vi "AlGaInPAs_v19b.vi"(2 "Debug Mode":bool, 3 "Elapsed Time(s)":dbl, 4 "State":enum16{"Edit", "Start", "Run", "End", "Idle"}(ring), 5 "Argument List In":string[](array[string])) -> (0 "Status Out":string, 1 "Argument List Out":string[](array[string]))   [LabVIEW 2011]
panel:
  out "In bubbler":T1 {"In main Copy"."Flow" format="%.2f"}
  out "Al bubbler":T2 {"Al main Copy"."Al Flow" format="%.2f"}
  out "P bubbler":T3 {"P bubbler main Copy"."Flow" format="%.2f"}
  out "As gas":T4 {"As gas main Copy"."Flow" format="%.2f"}
  out "P gas":T5 {"P gas main Copy"."Flow" format="%.2f"}
  out "Ga Bubbler":T6={"Ga main copy"={"Flow"=0.0, "Run"=FALSE, "Prep Ga"=FALSE, "Dilution"=FALSE}, "Ga MFC Flows copy"={"MFC2 flow"=10.0, "MFC3 flow"=100.0, "MFC1 flow"=1.0}, "Ga Calculated Copy"=1, "Ga bubbler Active"=FALSE} {"Ga Calculated Copy" items=["Ga flow", "MFC1", "MFC2", "MFC3"]; "Ga MFC Flows copy"."MFC1 flow" format="%.4f"; "Ga MFC Flows copy"."MFC3 flow" format="%.1f"; "Ga MFC Flows copy"."MFC2 flow" format="%.2f"; "Ga main copy"."Flow" format="%.2f"}
  in  "Al main":T7 caption="Al" {"Al Flow" format="%.2f"}
  in  "As gas main":T8 caption="Al" {"Flow" format="%.2f"}
  in  "P bubbler main":cluster{"Flow":dbl, "Run":bool, "Prep":bool} caption="Al" {"Flow" format="%.2f"}
  in  "P gas main":cluster{"Flow":dbl, "Run":bool, "Prep":bool} caption="Al" {"Flow" format="%.2f"}
  in  "In main":cluster{"Flow":dbl, "Run":bool, "Prep In":bool} caption="Al" {"Flow" format="%.2f"}
  out "prep_done":bool
  out "run started":bool
  out "first":bool=TRUE
  out "total time":dbl
  out "is OK?":bool
  in  "prep_time":dbl
  in  "Cancel":bool
  in  "OK":bool
  out "tTotal(s) 2":dbl
  in  "Ga Tab Control":enum32{"Page 1", "Page 2", "Page 3"}(tab)
  in  "Ga main":T9 caption="Al" {"Flow" format="%.2f"}
  in  "Ga MFC Flows":T10={"MFC2 flow"=10.0, "MFC3 flow"=100.0, "MFC1 flow"=1.0} {"MFC1 flow" format="%.4f"; "MFC3 flow" format="%.1f"; "MFC2 flow" format="%.2f"}
  in  "Ga Calculated":u16(ring)=1 caption="Calculated" items=["Ga flow", "MFC1", "MFC2", "MFC3"]
  # "Add pre-run time to run time in editor."
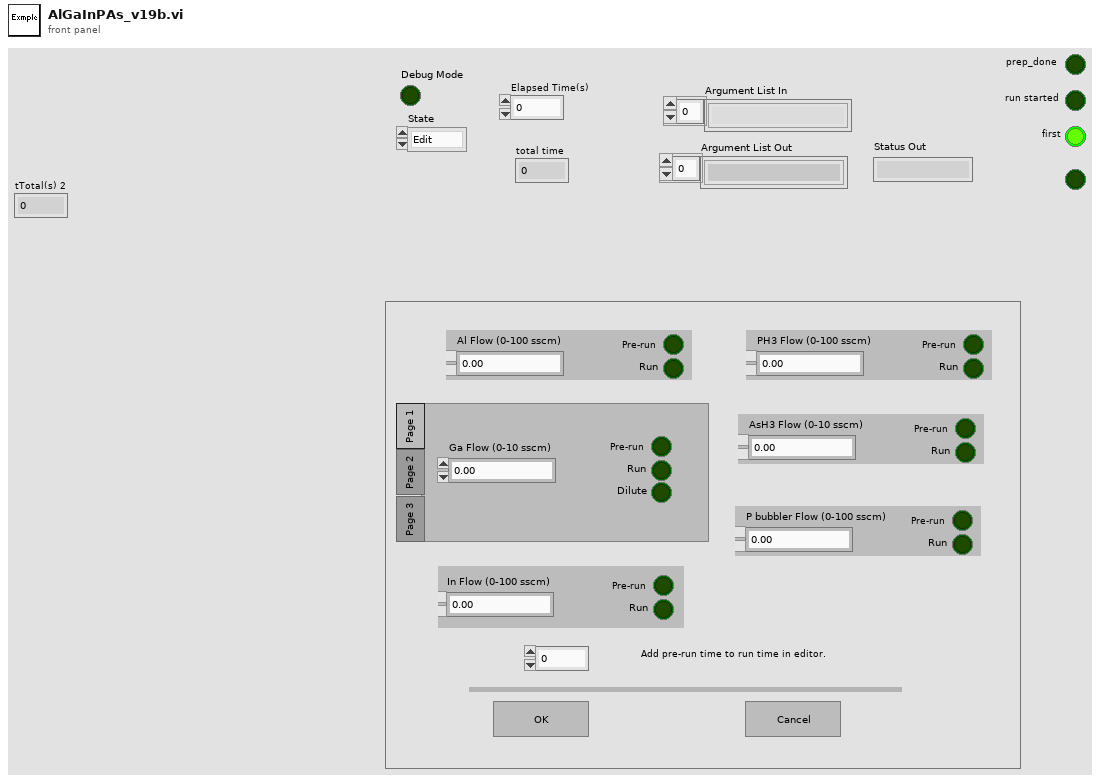
[diagram p1: front panel]
types:
  T1 = cluster{"In bubbler Active":bool, "In main Copy":cluster{"Flow":dbl, "Run":bool, "Prep In":bool}}
  T2 = cluster{"Al Active":bool, "Al main Copy":cluster{"Al Flow":dbl, "Al Run":bool, "Prep Al":bool}}
  T3 = cluster{"P bubbler Active":bool, "P bubbler main Copy":cluster{"Flow":dbl, "Run":bool, "Prep":bool}}
  T4 = cluster{"As gas Active":bool, "As gas main Copy":cluster{"Flow":dbl, "AsH3 Run":bool, "AsH3 Prep":bool}}
  T5 = cluster{"P gas Active":bool, "P gas main Copy":cluster{"Flow":dbl, "Run":bool, "Prep":bool}}
  T6 = cluster{"Ga main copy":cluster{"Flow":dbl, "Run":bool, "Prep Ga":bool, "Dilution":bool}, "Ga MFC Flows copy":cluster{"MFC2 flow":dbl, "MFC3 flow":dbl, "MFC1 flow":dbl}, "Ga Calculated Copy":u16, "Ga bubbler Active":bool}
  T7 = cluster{"Al Flow":dbl, "Al Run":bool, "Prep Al":bool}
  T8 = cluster{"Flow":dbl, "AsH3 Run":bool, "AsH3 Prep":bool}
  T9 = cluster{"Flow":dbl, "Run":bool, "Prep Ga":bool, "Dilution":bool}
  T10 = cluster{"MFC2 flow":dbl, "MFC3 flow":dbl, "MFC1 flow":dbl}
  T11 = enum16{"Discrete", "Continuous", "Instantaneous", "Finite"}
  T12 = enum32{"Invalid", "Default", "Floating", "Floating/Auto-Hide", "Modal"}
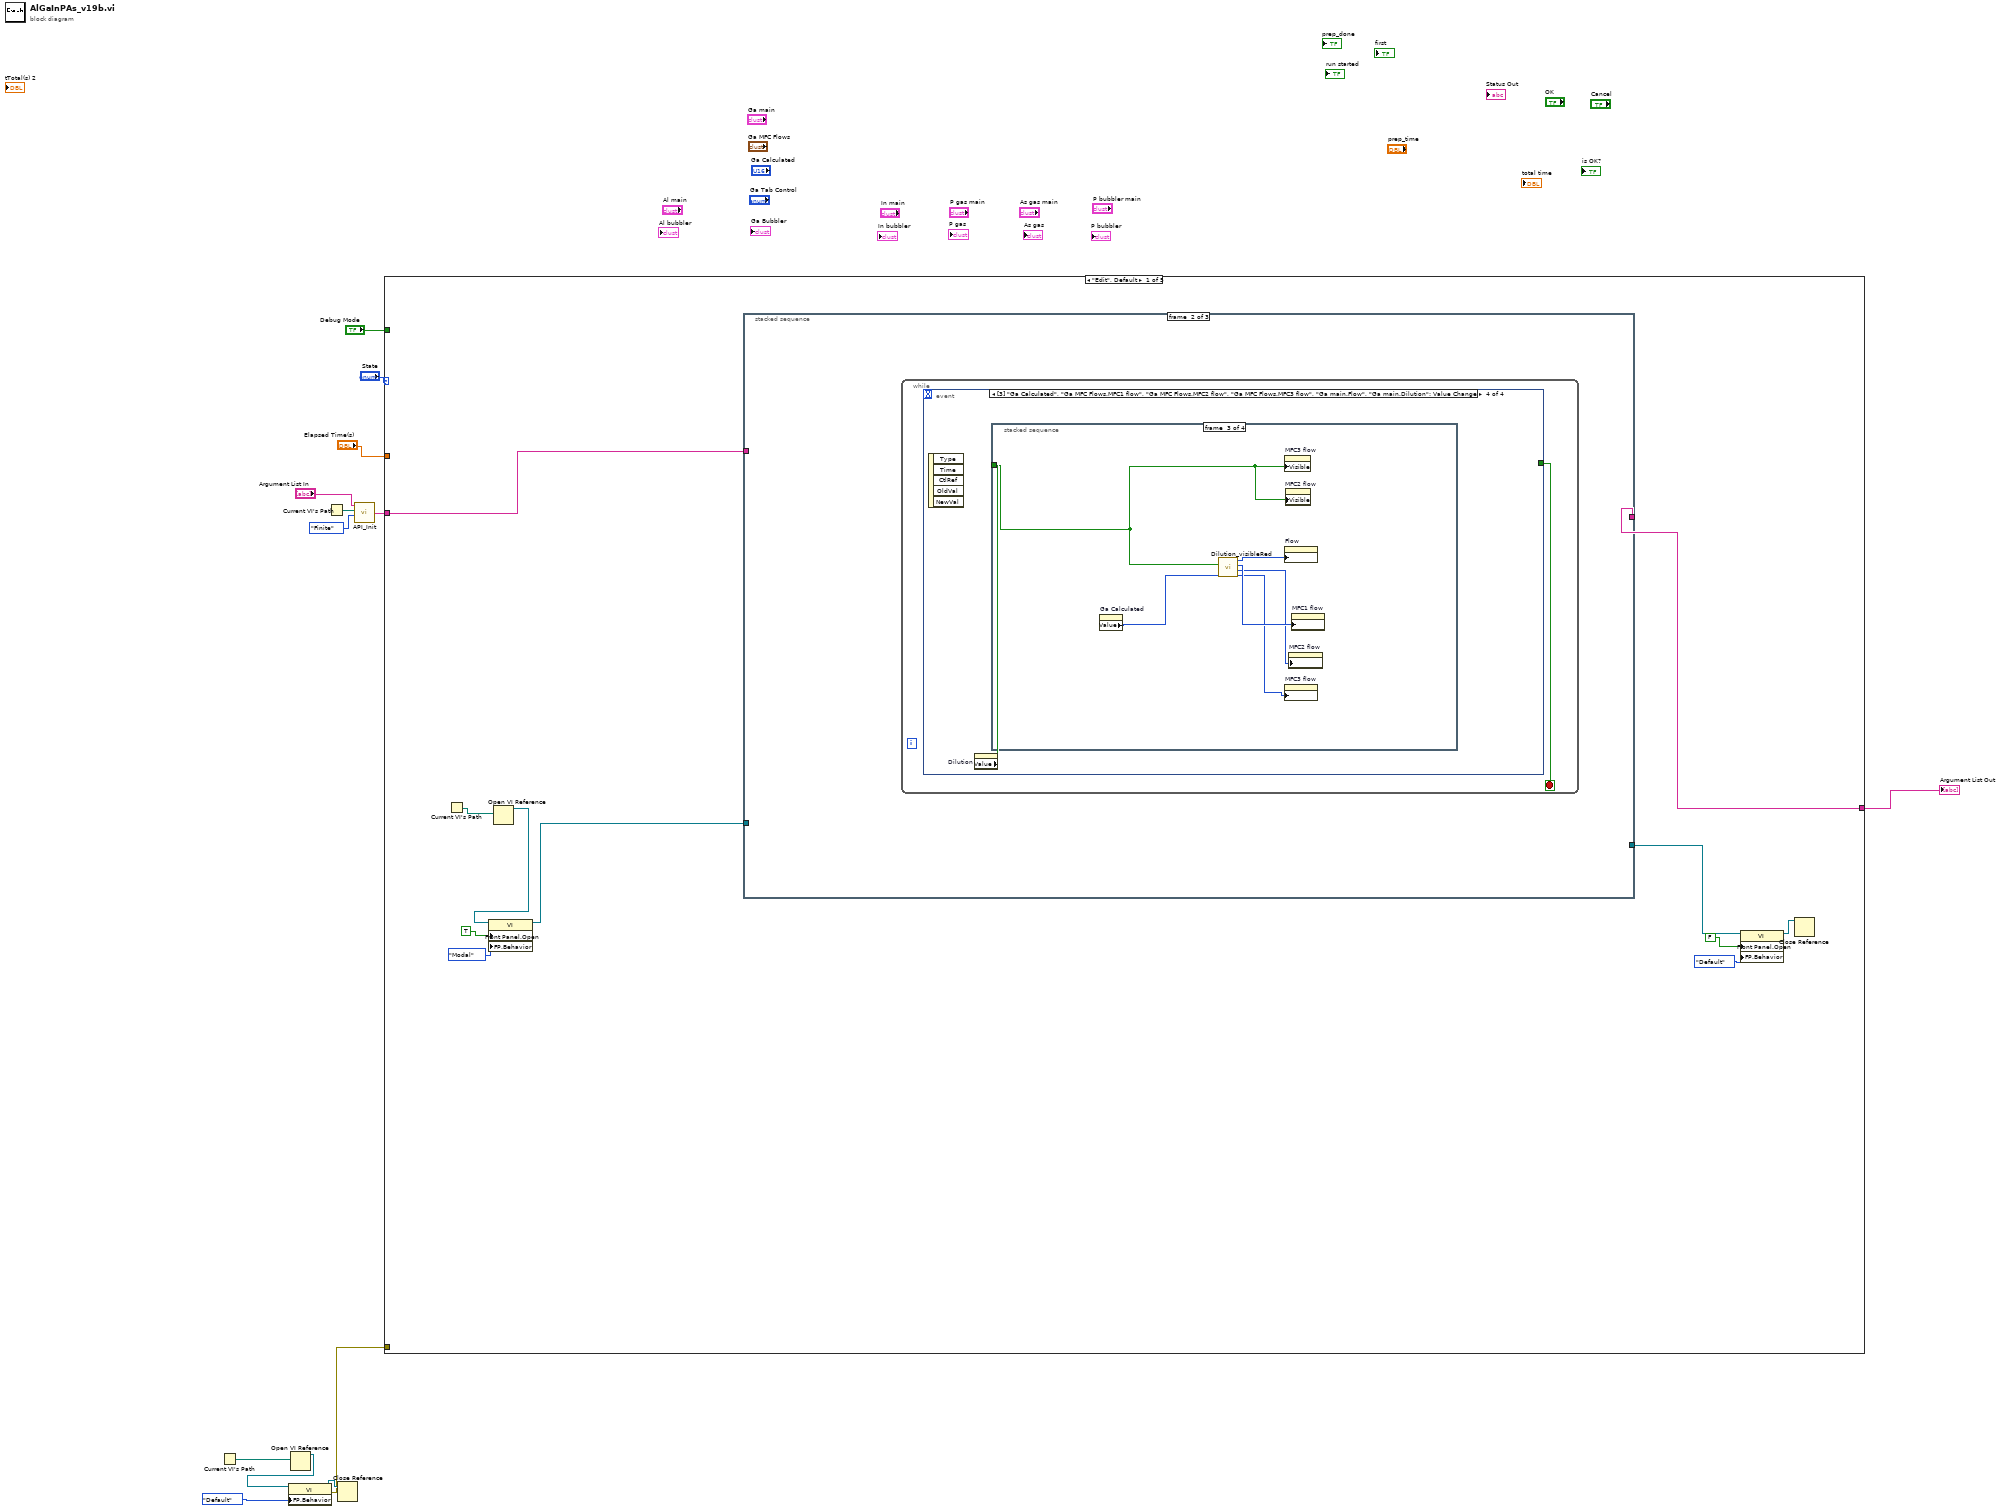
[diagram p0: block diagram]
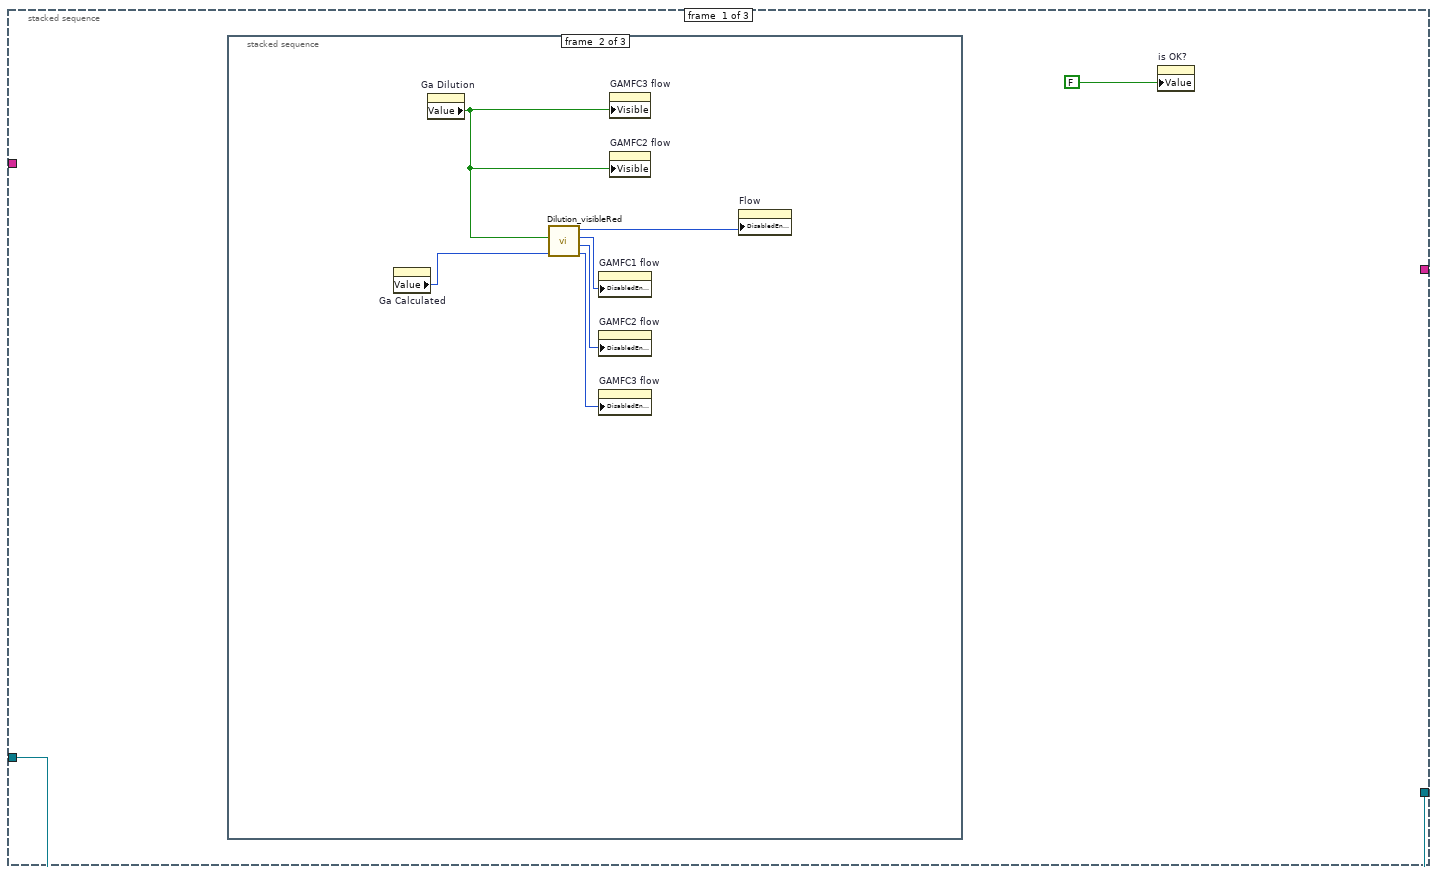
[diagram p2: hidden frame]
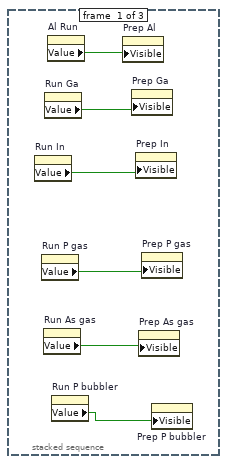
[diagram p3: hidden frame]
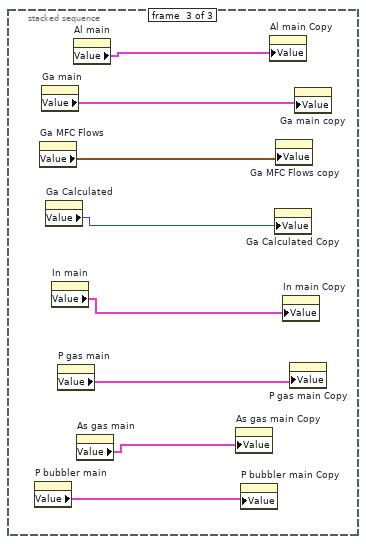
[diagram p4: hidden frame]
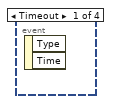
[diagram p5: hidden frame]
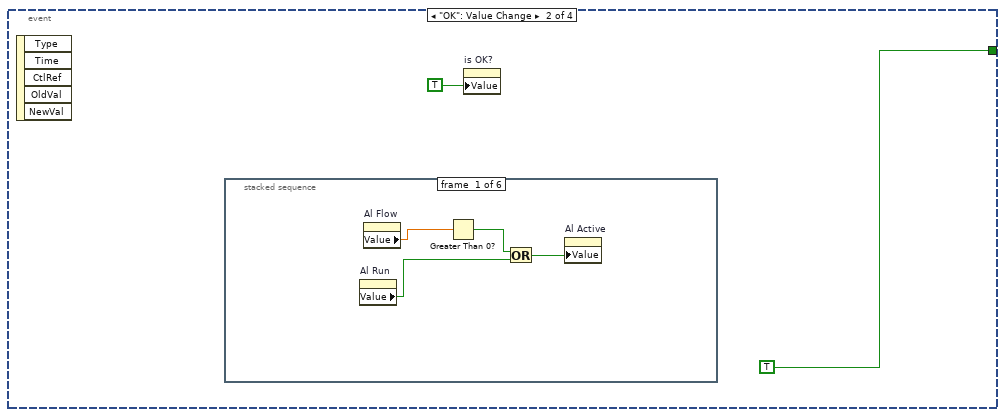
[diagram p6: hidden frame]
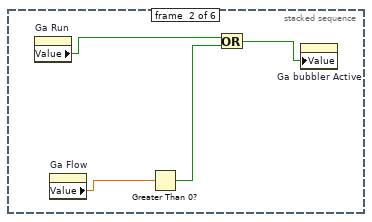
[diagram p7: hidden frame]
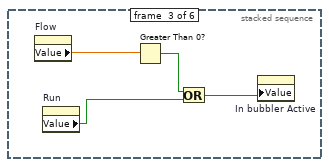
[diagram p8: hidden frame]
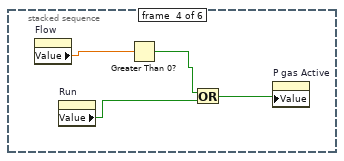
[diagram p9: hidden frame]
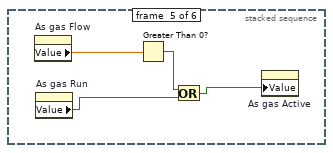
[diagram p10: hidden frame]
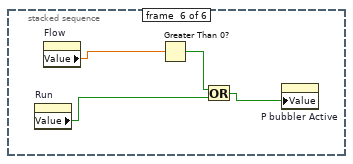
[diagram p11: hidden frame]
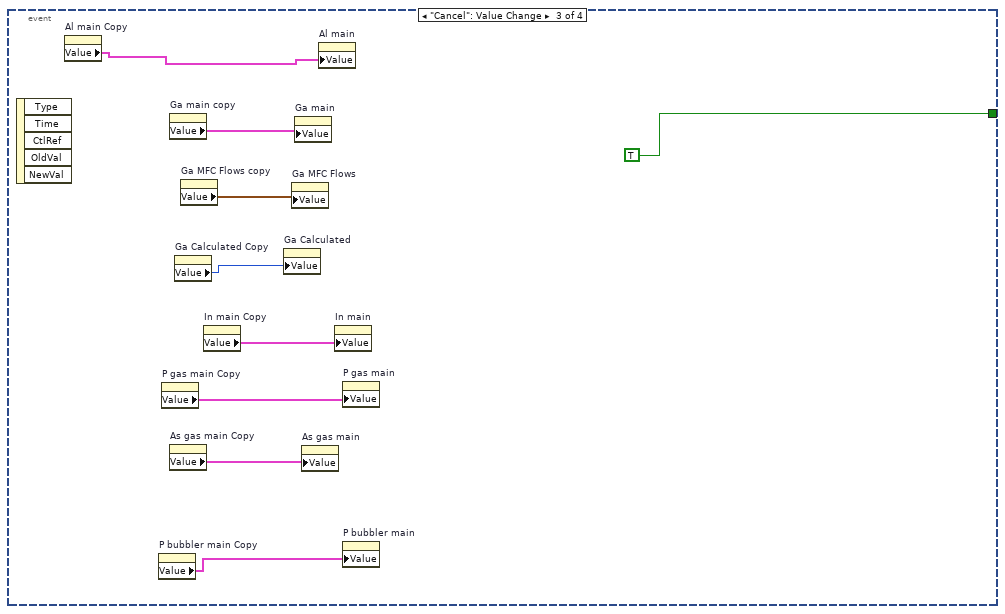
[diagram p12: hidden frame]
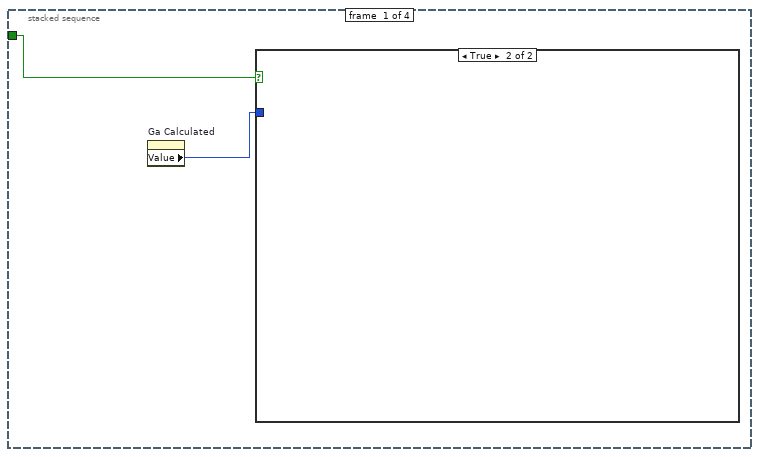
[diagram p13: hidden frame]
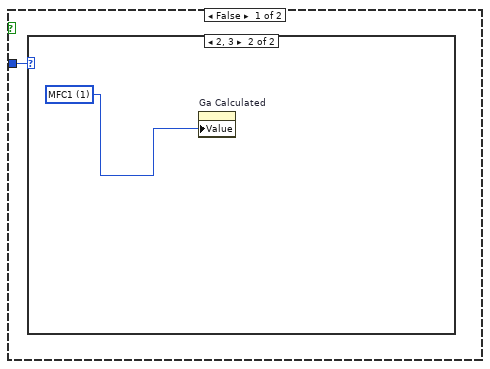
[diagram p14: hidden frame]
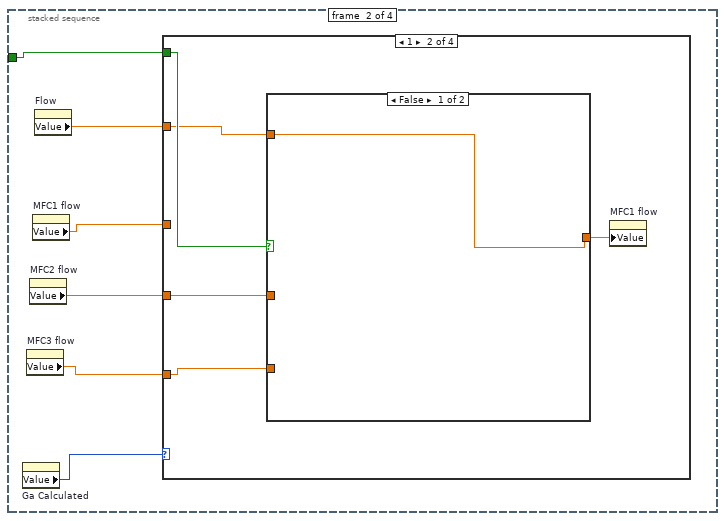
[diagram p16: hidden frame]
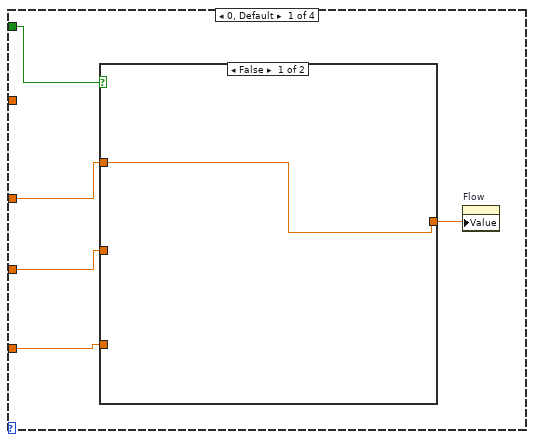
[diagram p17: hidden frame]
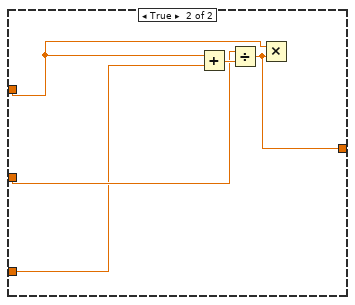
[diagram p18: hidden frame]
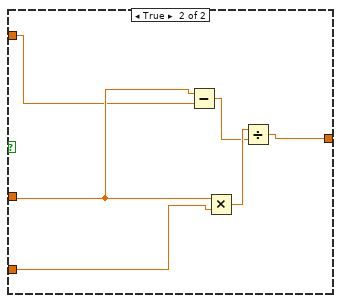
[diagram p19: hidden frame]
diagram:
  n1 = Current VI's Path() -> (path=w9:path)
  n2 = Open VI Reference(vi path=w9) -> (vi reference=w8:refnum<vi>)  [unwired: 1 in, 5 out]
  n3 = property class="VI"(reference=w8, "FP.Behavior"=T12."Default" ("Front Panel Window:Behavior")) -> (reference out=w6:refnum<vi>, error out=w5:errorcluster)  [unwired: 1 in]
  n4 = Current VI's Path() -> (path=w4:path)
  n5 = Close Reference(reference=w6) -> ()  [unwired: 1 in, 1 out]
  n6 = call "API_Init.vi"("API Mode"=T11."Finite", "VI Path"=w4, "Argument List In"="Argument List In") -> ("Argument List Out"=w1:string[])  [unwired: 1 in]
  n7 = case shown="\"Edit\", Default" "State" {
    tunnel: "Debug Mode" -> [_ w151 w209 _ _]
    tunnel: "Elapsed Time(s)" -> [_ _ w210 _ _]
    tunnel: w1 -> [w15 w153 w208 w314 w315]
    tunnel: [w14 w152 w207 w314 w315] -> w10
    tunnel: w5 -> [_ _ _ _ _]
    frame "Edit", Default {
      n8 = Current VI's Path() -> (path=w20:path)
      n9 = Open VI Reference(vi path=w20) -> (vi reference=w19:refnum<vi>)  [unwired: 1 in, 5 out]
      n10 = property class="VI"(reference=w19, "Front Panel.Open"=TRUE ("Front Panel Window:Open"), "FP.Behavior"=T12."Modal" ("Front Panel Window:Behavior")) -> (reference out=w18:refnum<vi>)  [unwired: 1 in, 1 out]
      n11 = stacked-sequence {
        tunnel: w15 -> [_ _ w147]
        tunnel: w18 -> [w26 _ _]
        tunnel: [w26 _ _] -> w22
        tunnel: [_ _ w148] -> w14
        frame #0 {
          n12 = stacked-sequence {
            frame #0 {
              n13 = property on="Run In" class="Bool (strict)"() -> ("Value"=w31:bool)  [unwired: 2 in, 2 out]
              n14 = property on="Run P gas" class="Bool (strict)"() -> ("Value"=w29:bool)  [unwired: 2 in, 2 out]
              n15 = property on="Run As gas" class="Bool (strict)"() -> ("Value"=w28:bool)  [unwired: 2 in, 2 out]
              n16 = property on="Run Ga" class="Bool (strict)"() -> ("Value"=w30:bool)  [unwired: 2 in, 2 out]
              n17 = property on="Al Run" class="Bool (strict)"() -> ("Value"=w32:bool)  [unwired: 2 in, 2 out]
              n18 = property on="Run P bubbler" class="Bool (strict)"() -> ("Value"=w27:bool)  [unwired: 2 in, 2 out]
              n19 = property on="Prep Al" class="Bool (strict)"("Visible"=w32) -> ()  [unwired: 2 in, 2 out]
              n20 = property on="Prep Ga" class="Bool (strict)"("Visible"=w30) -> ()  [unwired: 2 in, 2 out]
              n21 = property on="Prep In" class="Bool (strict)"("Visible"=w31) -> ()  [unwired: 2 in, 2 out]
              n22 = property on="Prep As gas" class="Bool (strict)"("Visible"=w28) -> ()  [unwired: 2 in, 2 out]
              n23 = property on="Prep P gas" class="Bool (strict)"("Visible"=w29) -> ()  [unwired: 2 in, 2 out]
              n24 = property on="Prep P bubbler" class="Bool (strict)"("Visible"=w27) -> ()  [unwired: 2 in, 2 out]
            }
            frame #1 {
              n25 = property on="Ga Calculated" class="Ring (strict)"() -> ("Value"=w38:u16)  [unwired: 2 in, 2 out]
              n26 = property on="Ga Dilution" class="Bool (strict)"() -> ("Value"=w37:bool)  [unwired: 2 in, 2 out]
              n27 = call "Dilution_visibleRed.vi"("calculated"=w38, "dilution"=w37) -> ("MFC3"=w34:u16, "MFC2"=w35:u16, "MFC1"=w36:u16, "flow"=w33:u16)  [unwired: 2 in]
              n28 = property on="GAMFC1 flow" class="DigNum (strict)"("DisabledEnum"=w36) -> ()  [unwired: 2 in, 2 out]
              n29 = property on="GAMFC2 flow" class="DigNum (strict)"("DisabledEnum"=w35) -> ()  [unwired: 2 in, 2 out]
              n30 = property on="GAMFC3 flow" class="DigNum (strict)"("DisabledEnum"=w34) -> ()  [unwired: 2 in, 2 out]
              n31 = property on="GAMFC3 flow" class="DigNum (strict)"("Visible"=w37) -> ()  [unwired: 2 in, 2 out]
              n32 = property on="GAMFC2 flow" class="DigNum (strict)"("Visible"=w37) -> ()  [unwired: 2 in, 2 out]
              n33 = property on="Flow" class="DigNum (strict)"("DisabledEnum"=w33) -> ()  [unwired: 2 in, 2 out]
            }
            frame #2 {
              n34 = property on="P bubbler main" class="Clust (strict)"() -> ("Value"=w40:cluster{"Flow":dbl, "Run":bool, "Prep":bool})  [unwired: 2 in, 2 out]
              n35 = property on="Ga MFC Flows" class="Clust (strict)"() -> ("Value"=w45:T10)  [unwired: 2 in, 2 out]
              n36 = property on="Ga main" class="Clust (strict)"() -> ("Value"=w46:T9)  [unwired: 2 in, 2 out]
              n37 = property on="Ga Calculated" class="Ring (strict)"() -> ("Value"=w44:u16)  [unwired: 2 in, 2 out]
              n38 = property on="In main" class="Clust (strict)"() -> ("Value"=w43:cluster{"Flow":dbl, "Run":bool, "Prep In":bool})  [unwired: 2 in, 2 out]
              n39 = property on="P gas main" class="Clust (strict)"() -> ("Value"=w42:cluster{"Flow":dbl, "Run":bool, "Prep":bool})  [unwired: 2 in, 2 out]
              n40 = property on="Al main" class="Clust (strict)"() -> ("Value"=w39:T7)  [unwired: 2 in, 2 out]
              n41 = property on="As gas main" class="Clust (strict)"() -> ("Value"=w41:T8)  [unwired: 2 in, 2 out]
              n42 = property on="As gas main Copy" class="Clust (strict)"("Value"=w41) -> ()  [unwired: 2 in, 2 out]
              n43 = property on="P bubbler main Copy" class="Clust (strict)"("Value"=w40) -> ()  [unwired: 2 in, 2 out]
              n44 = property on="Al main Copy" class="Clust (strict)"("Value"=w39) -> ()  [unwired: 2 in, 2 out]
              n45 = property on="Ga Calculated Copy" class="Ring (strict)"("Value"=w44) -> ()  [unwired: 2 in, 2 out]
              n46 = property on="Ga MFC Flows copy" class="Clust (strict)"("Value"=w45) -> ()  [unwired: 2 in, 2 out]
              n47 = property on="In main Copy" class="Clust (strict)"("Value"=w43) -> ()  [unwired: 2 in, 2 out]
              n48 = property on="P gas main Copy" class="Clust (strict)"("Value"=w42) -> ()  [unwired: 2 in, 2 out]
              n49 = property on="Ga main copy" class="Clust (strict)"("Value"=w46) -> ()  [unwired: 2 in, 2 out]
            }
          }
          n50 = property on="is OK?" class="Bool (strict)"("Value"=FALSE ("is OK?")) -> ()  [unwired: 2 in, 2 out]
        }
        frame #1 {
          n51 = while {
            stop <- w47 stop-if-true
            n52 = event shown="[3] \"Ga Calculated\", \"Ga MFC Flows.MFC1 flow\", \"Ga MFC Flows.MFC2 flow\", \"Ga MFC Flows.MFC3 flow\", \"Ga main.Flow\", \"Ga main.Dilution\": Value Change" {
              selector: _ -> [_ _ _ _]
              dyn-events: _ -> [_ _ _ _]
              timeout: _ -> [_ _ _ _]
              tunnel: [_ TRUE TRUE _] -> w47
              event Timeout {
                n53 = event-data() -> ()  [unwired: 1 in, 2 out]
              }
              event "OK": Value Change {
                n54 = event-data() -> ()  [unwired: 1 in, 5 out]
                n55 = stacked-sequence {
                  frame #0 {
                    n56 = property on="Al Run" class="Bool (strict)"() -> ("Value"=w51:bool)  [unwired: 2 in, 2 out]
                    n57 = property on="Al Flow" class="DigNum (strict)"() -> ("Value"=w52:dbl)  [unwired: 2 in, 2 out]
                    n58 = Greater Than 0?(x=w52) -> (x > 0?=w53:bool)
                    n59 = Or(x=w53, y=w51) -> (x .or. y?=w50:bool)
                    n60 = property on="Al Active" class="Bool (strict)"("Value"=w50) -> ()  [unwired: 2 in, 2 out]
                  }
                  frame #1 {
                    n61 = property on="Ga Run" class="Bool (strict)"() -> ("Value"=w55:bool)  [unwired: 2 in, 2 out]
                    n62 = property on="Ga Flow" class="DigNum (strict)"() -> ("Value"=w54:dbl)  [unwired: 2 in, 2 out]
                    n63 = Greater Than 0?(x=w54) -> (x > 0?=w57:bool)
                    n64 = Or(x=w55, y=w57) -> (x .or. y?=w56:bool)
                    n65 = property on="Ga bubbler Active" class="Bool (strict)"("Value"=w56) -> ()  [unwired: 2 in, 2 out]
                  }
                  frame #2 {
                    n66 = property on="Flow" class="DigNum (strict)"() -> ("Value"=w60:dbl)  [unwired: 2 in, 2 out]
                    n67 = property on="Run" class="Bool (strict)"() -> ("Value"=w59:bool)  [unwired: 2 in, 2 out]
                    n68 = Greater Than 0?(x=w60) -> (x > 0?=w61:bool)
                    n69 = Or(x=w61, y=w59) -> (x .or. y?=w58:bool)
                    n70 = property on="In bubbler Active" class="Bool (strict)"("Value"=w58) -> ()  [unwired: 2 in, 2 out]
                  }
                  frame #3 {
                    n71 = property on="Flow" class="DigNum (strict)"() -> ("Value"=w64:dbl)  [unwired: 2 in, 2 out]
                    n72 = property on="Run" class="Bool (strict)"() -> ("Value"=w63:bool)  [unwired: 2 in, 2 out]
                    n73 = Greater Than 0?(x=w64) -> (x > 0?=w65:bool)
                    n74 = Or(x=w65, y=w63) -> (x .or. y?=w62:bool)
                    n75 = property on="P gas Active" class="Bool (strict)"("Value"=w62) -> ()  [unwired: 2 in, 2 out]
                  }
                  frame #4 {
                    n76 = property on="As gas Flow" class="DigNum (strict)"() -> ("Value"=w68:dbl)  [unwired: 2 in, 2 out]
                    n77 = property on="As gas Run" class="Bool (strict)"() -> ("Value"=w67:bool)  [unwired: 2 in, 2 out]
                    n78 = Greater Than 0?(x=w68) -> (x > 0?=w69:bool)
                    n79 = Or(x=w69, y=w67) -> (x .or. y?=w66:bool)
                    n80 = property on="As gas Active" class="Bool (strict)"("Value"=w66) -> ()  [unwired: 2 in, 2 out]
                  }
                  frame #5 {
                    n81 = property on="Run" class="Bool (strict)"() -> ("Value"=w71:bool)  [unwired: 2 in, 2 out]
                    n82 = property on="Flow" class="DigNum (strict)"() -> ("Value"=w72:dbl)  [unwired: 2 in, 2 out]
                    n83 = Greater Than 0?(x=w72) -> (x > 0?=w73:bool)
                    n84 = Or(x=w73, y=w71) -> (x .or. y?=w70:bool)
                    n85 = property on="P bubbler Active" class="Bool (strict)"("Value"=w70) -> ()  [unwired: 2 in, 2 out]
                  }
                }
                n86 = property on="is OK?" class="Bool (strict)"("Value"=TRUE ("is OK?")) -> ()  [unwired: 2 in, 2 out]
              }
              event "Cancel": Value Change {
                n87 = event-data() -> ()  [unwired: 1 in, 5 out]
                n88 = property on="Al main Copy" class="Clust (strict)"() -> ("Value"=w74:T7)  [unwired: 2 in, 2 out]
                n89 = property on="P bubbler main Copy" class="Clust (strict)"() -> ("Value"=w75:cluster{"Flow":dbl, "Run":bool, "Prep":bool})  [unwired: 2 in, 2 out]
                n90 = property on="P gas main Copy" class="Clust (strict)"() -> ("Value"=w80:cluster{"Flow":dbl, "Run":bool, "Prep":bool})  [unwired: 2 in, 2 out]
                n91 = property on="Ga main copy" class="Clust (strict)"() -> ("Value"=w79:T9)  [unwired: 2 in, 2 out]
                n92 = property on="As gas main Copy" class="Clust (strict)"() -> ("Value"=w76:T8)  [unwired: 2 in, 2 out]
                n93 = property on="Ga Calculated Copy" class="Ring (strict)"() -> ("Value"=w77:u16)  [unwired: 2 in, 2 out]
                n94 = property on="Ga MFC Flows copy" class="Clust (strict)"() -> ("Value"=w78:T10)  [unwired: 2 in, 2 out]
                n95 = property on="In main Copy" class="Clust (strict)"() -> ("Value"=w81:cluster{"Flow":dbl, "Run":bool, "Prep In":bool})  [unwired: 2 in, 2 out]
                n96 = property on="Ga Calculated" class="Ring (strict)"("Value"=w77) -> ()  [unwired: 2 in, 2 out]
                n97 = property on="Ga MFC Flows" class="Clust (strict)"("Value"=w78) -> ()  [unwired: 2 in, 2 out]
                n98 = property on="Ga main" class="Clust (strict)"("Value"=w79) -> ()  [unwired: 2 in, 2 out]
                n99 = property on="As gas main" class="Clust (strict)"("Value"=w76) -> ()  [unwired: 2 in, 2 out]
                n100 = property on="Al main" class="Clust (strict)"("Value"=w74) -> ()  [unwired: 2 in, 2 out]
                n101 = property on="In main" class="Clust (strict)"("Value"=w81) -> ()  [unwired: 2 in, 2 out]
                n102 = property on="P gas main" class="Clust (strict)"("Value"=w80) -> ()  [unwired: 2 in, 2 out]
                n103 = property on="P bubbler main" class="Clust (strict)"("Value"=w75) -> ()  [unwired: 2 in, 2 out]
              }
              event "Ga Calculated", "Ga MFC Flows.MFC1 flow", "Ga MFC Flows.MFC2 flow", "Ga MFC Flows.MFC3 flow", "Ga main.Flow", "Ga main.Dilution": Value Change {
                n104 = event-data() -> ()  [unwired: 1 in, 5 out]
                n105 = property on="Dilution" class="Bool (strict)"() -> ("Value"=w83:bool)  [unwired: 2 in, 2 out]
                n106 = stacked-sequence {
                  tunnel: w83 -> [w84 w92 w137 w143]
                  frame #0 {
                    n107 = property on="Ga Calculated" class="Ring (strict)"() -> ("Value"=w85:u16)  [unwired: 2 in, 2 out]
                    n108 = case shown="True" w84 {
                      tunnel: w85 -> [w86 _]
                      frame False {
                        n109 = case shown="2, 3" w86 {
                          frame 0, 1, Default {
                          }
                          frame 2, 3 {
                            w87 = u16 1 items=["Ga flow", "MFC1", "MFC2", "MFC3"] ("Ga calculated")
                            n110 = property on="Ga Calculated" class="Ring (strict)"("Value"=w87) -> ()  [unwired: 2 in, 2 out]
                          }
                        }
                      }
                      frame True {
                      }
                    }
                  }
                  frame #1 {
                    n111 = property on="Ga Calculated" class="Ring (strict)"() -> ("Value"=w93:u16)  [unwired: 2 in, 2 out]
                    n112 = property on="MFC3 flow" class="DigNum (strict)"() -> ("Value"=w89:dbl)  [unwired: 2 in, 2 out]
                    n113 = property on="MFC2 flow" class="DigNum (strict)"() -> ("Value"=w90:dbl)  [unwired: 2 in, 2 out]
                    n114 = property on="MFC1 flow" class="DigNum (strict)"() -> ("Value"=w91:dbl)  [unwired: 2 in, 2 out]
                    n115 = property on="Flow" class="DigNum (strict)"() -> ("Value"=w88:dbl)  [unwired: 2 in, 2 out]
                    n116 = case shown="1" w93 {
                      tunnel: w92 -> [w98 w109 w120 w130]
                      tunnel: w91 -> [w97 _ w119 w129]
                      tunnel: w90 -> [w96 w106 _ w127]
                      tunnel: w89 -> [w95 w105 w118 _]
                      tunnel: w88 -> [_ w108 w117 w128]
                      frame 0, Default {
                        n117 = case shown="False" w98 {
                          tunnel: w97 -> [w99 w103]
                          tunnel: w96 -> [_ w102]
                          tunnel: w95 -> [_ w101]
                          tunnel: [w99 w100] -> w94
                          frame False {
                          }
                          frame True {
                            n118 = Add(x=w103, y=w101) -> (x+y=w104:dbl)
                            n119 = Divide(x=w102, y=w104) -> (x/y=w100:dbl)
                            n120 = Multiply(x=w103, y=w100) -> ()  [unwired: 1 out]
                          }
                        }
                        n121 = property on="Flow" class="DigNum (strict)"("Value"=w94) -> ()  [unwired: 2 in, 2 out]
                      }
                      frame 1 {
                        n122 = case shown="False" w109 {
                          tunnel: w108 -> [w110 w112]
                          tunnel: [w110 w111] -> w107
                          tunnel: w106 -> [_ w114]
                          tunnel: w105 -> [_ w113]
                          frame False {
                          }
                          frame True {
                            n123 = Subtract(x=w114, y=w112) -> (x-y=w115:dbl)
                            n124 = Multiply(x=w114, y=w113) -> (x*y=w116:dbl)
                            n125 = Divide(x=w116, y=w115) -> (x/y=w111:dbl)
                          }
                        }
                        n126 = property on="MFC1 flow" class="DigNum (strict)"("Value"=w107) -> ()  [unwired: 2 in, 2 out]
                      }
                      frame 2 {
                        n127 = case shown="False" w120 {
                          tunnel: w119 -> [_ w122]
                          tunnel: w118 -> [_ w124]
                          tunnel: w117 -> [_ w123]
                          frame False {
                          }
                          frame True {
                            n128 = Add(x=w122, y=w124) -> (x+y=w126:dbl)
                            n129 = Multiply(x=w123, y=w126) -> (x*y=w125:dbl)
                            n130 = Divide(x=w125, y=w122) -> (x/y=w121:dbl)
                            n131 = property on="MFC2 flow" class="DigNum (strict)"("Value"=w121) -> ()  [unwired: 2 in, 2 out]
                          }
                        }
                      }
                      frame 3 {
                        n132 = case shown="False" w130 {
                          tunnel: w129 -> [_ w134]
                          tunnel: w128 -> [_ w133]
                          tunnel: w127 -> [_ w132]
                          frame False {
                          }
                          frame True {
                            n133 = Subtract(x=w132, y=w133) -> (x-y=w135:dbl)
                            n134 = Divide(x=w134, y=w133) -> (x/y=w136:dbl)
                            n135 = Multiply(x=w136, y=w135) -> (x*y=w131:dbl)
                            n136 = property on="MFC3 flow" class="DigNum (strict)"("Value"=w131) -> ()  [unwired: 2 in, 2 out]
                          }
                        }
                      }
                    }
                  }
                  frame #2 {
                    n137 = property on="Ga Calculated" class="Ring (strict)"() -> ("Value"=w142:u16)  [unwired: 2 in, 2 out]
                    n138 = call "Dilution_visibleRed.vi"("calculated"=w142, "dilution"=w137) -> ("MFC3"=w138:u16, "MFC2"=w139:u16, "MFC1"=w140:u16, "flow"=w141:u16)  [unwired: 2 in]
                    n139 = property on="MFC3 flow" class="DigNum (strict)"("Visible"=w137) -> ()  [unwired: 2 in, 2 out]
                    n140 = property on="Flow" class="DigNum (strict)"("DisabledEnum"=w141) -> ()  [unwired: 2 in, 2 out]
                    n141 = property on="MFC3 flow" class="DigNum (strict)"("DisabledEnum"=w138) -> ()  [unwired: 2 in, 2 out]
                    n142 = property on="MFC2 flow" class="DigNum (strict)"("Visible"=w137) -> ()  [unwired: 2 in, 2 out]
                    n143 = property on="MFC2 flow" class="DigNum (strict)"("DisabledEnum"=w139) -> ()  [unwired: 2 in, 2 out]
                    n144 = property on="MFC1 flow" class="DigNum (strict)"("DisabledEnum"=w140) -> ()  [unwired: 2 in, 2 out]
                  }
                  frame #3 {
                    n145 = case shown="True" w143 {
                      frame False {
                        n146 = property on="Ga Calculated" class="Ring (strict)"("Disabled Items []"=i32[] [2, 3]) -> ()  [unwired: 2 in, 2 out]
                      }
                      frame True {
                        n147 = property on="Ga Calculated" class="Ring (strict)"("Disabled Items []"=i32[] []) -> ()  [unwired: 2 in, 2 out]
                      }
                    }
                  }
                }
              }
            }
          }
        }
        frame #2 {
          n148 = property on="is OK?" class="Bool (strict)"() -> ("Value"=w146:bool)  [unwired: 2 in, 2 out]
          n149 = Not(x=w146) -> (.not. x?=w150:bool)
          n150 = Current VI's Path() -> (path=w149:path)
          n151 = call "API_Edit.vi"("Cancel"=w150, "OK"=w146, "VI Path"=w149, "Argument List In"=w147) -> ("Argument List Out"=w148:string[])
        }
      }
      n152 = property class="VI"(reference=w22, "Front Panel.Open"=FALSE ("Front Panel Window:Open"), "FP.Behavior"=T12."Default" ("Front Panel Window:Behavior")) -> (reference out=w23:refnum<vi>)  [unwired: 1 in, 1 out]
      n153 = Close Reference(reference=w23) -> ()  [unwired: 1 in, 1 out]
    }
    frame "Start" {
      n154 = call "Set_Argument.vi"("Enable"=FALSE, "Argument"="run_started", "Argument List In"=w153) -> ("Argument List Out"=w152:string[])
      n155 = case shown="False" w151 {
        frame False {
          n156 = stacked-sequence {
            frame #0 {
              n157 = property on="Al Active" class="Bool (strict)"() -> ("Value"=w156:bool)  [unwired: 2 in, 2 out]
              n158 = case shown="True" w156 {
                frame False {
                  w157 = FALSE ("Al Active")
                  n159 = call "set_Al.vi"("ALMFC1"=0.0 ("Aluminum Flow"), "Remote"=w157, "Run"=w157, "Bubbler In"=w157, "Active"=w157) -> ()  [unwired: 5 out]
                }
                frame True {
                  w163 = TRUE ("Al Active")
                  n160 = property on="Al Run" class="Bool (strict)"() -> ("Value"=w159:bool)  [unwired: 2 in, 2 out]
                  n161 = property on="Prep Al" class="Bool (strict)"() -> ("Value"=w160:bool)  [unwired: 2 in, 2 out]
                  n162 = And(x=w160, y=w159) -> (x .and. y?=w162:bool)
                  n163 = property on="Al Flow" class="DigNum (strict)"() -> ("Value"=w161:dbl)  [unwired: 2 in, 2 out]
                  n164 = call "set_Al.vi"("ALMFC1"=w161, "Run"=w162, "Bubbler In"=w163, "Active"=w163) -> ()  [unwired: 1 in, 5 out]
                }
              }
            }
            frame #1 {
              n165 = property on="Ga bubbler Active" class="Bool (strict)"() -> ("Value"=w164:bool)  [unwired: 2 in, 2 out]
              n166 = case shown="True" w164 {
                frame False {
                  w166 = FALSE ("Ga Active")
                  w165 = 0.0 ("Ga Flow 1")
                  n167 = call "set_Ga.vi"("Active"=w166, "GAMFC3"=w165, "GAMFC2"=w165, "GAMFC1"=w165, "Bubbler In"=w166, "H2 Dilute"=w166, "Run"=w166, "Remote"=w166) -> ()  [unwired: 8 out]
                }
                frame True {
                  w173 = TRUE ("Ga Active")
                  n168 = property on="Prep Ga" class="Bool (strict)"() -> ("Value"=w170:bool)  [unwired: 2 in, 2 out]
                  n169 = property on="Dilution" class="Bool (strict)"() -> ("Value"=w172:bool)  [unwired: 2 in, 2 out]
                  n170 = property on="MFC1 flow" class="DigNum (strict)"() -> ("Value"=w169:dbl)  [unwired: 2 in, 2 out]
                  n171 = property on="Run" class="Bool (strict)"() -> ("Value"=w171:bool)  [unwired: 2 in, 2 out]
                  n172 = And(x=w170, y=w171) -> (x .and. y?=w174:bool)
                  n173 = property on="MFC2 flow" class="DigNum (strict)"() -> ("Value"=w168:dbl)  [unwired: 2 in, 2 out]
                  n174 = property on="MFC3 flow" class="DigNum (strict)"() -> ("Value"=w167:dbl)  [unwired: 2 in, 2 out]
                  n175 = call "set_Ga.vi"("Active"=w173, "GAMFC3"=w167, "GAMFC2"=w168, "GAMFC1"=w169, "Bubbler In"=w173, "H2 Dilute"=w172, "Run"=w174, "Remote"=w173) -> ()  [unwired: 8 in]
                }
              }
            }
            frame #2 {
              n176 = property on="In bubbler Active" class="Bool (strict)"() -> ("Value"=w175:bool)  [unwired: 2 in, 2 out]
              n177 = case shown="False" w175 {
                frame False {
                  w177 = FALSE ("In Remote")
                  n178 = call "set_In.vi"("INMFC1"=0.0 ("Indium Flow"), "Remote"=w177, "Run"=w177, "Bubbler In"=w177, "Active"=w177) -> ()  [unwired: 5 out]
                }
                frame True {
                  w182 = TRUE ("In Run")
                  n179 = property on="Run" class="Bool (strict)"() -> ("Value"=w179:bool)  [unwired: 2 in, 2 out]
                  n180 = property on="Prep In" class="Bool (strict)"() -> ("Value"=w180:bool)  [unwired: 2 in, 2 out]
                  n181 = And(x=w179, y=w180) -> (x .and. y?=w181:bool)
                  n182 = property on="Flow" class="DigNum (strict)"() -> ("Value"=w178:dbl)  [unwired: 2 in, 2 out]
                  n183 = call "set_In.vi"("INMFC1"=w178, "Run"=w181, "Bubbler In"=w182, "Active"=w182) -> ()  [unwired: 1 in, 5 out]
                }
              }
            }
            frame #3 {
              n184 = property on="P gas Active" class="Bool (strict)"() -> ("Value"=w183:bool)  [unwired: 2 in, 2 out]
              n185 = case shown="False" w183 {
                frame False {
                  w184 = FALSE ("P_Gas Active")
                  n186 = call "set_P_gas.vi"("Run"=w184, "Gas In"=w184, "Active"=w184, "P_Gas Remote"=w184, "H2 Flush"=w184, "P_Gas Flow"=0.0) -> ()
                }
                frame True {
                  w190 = TRUE ("P_Gas Active")
                  n187 = property on="Flow" class="DigNum (strict)"() -> ("Value"=w188:dbl)  [unwired: 2 in, 2 out]
                  n188 = property on="Prep" class="Bool (strict)"() -> ("Value"=w187:bool)  [unwired: 2 in, 2 out]
                  n189 = property on="Run" class="Bool (strict)"() -> ("Value"=w186:bool)  [unwired: 2 in, 2 out]
                  n190 = And(x=w187, y=w186) -> (x .and. y?=w189:bool)
                  n191 = call "set_P_gas.vi"("Active"=w190, "P_Gas Remote"=w189, "H2 Flush"=w190, "P_Gas Flow"=w188) -> ()  [unwired: 2 in]
                }
              }
            }
            frame #4 {
              n192 = property on="As gas Active" class="Bool (strict)"() -> ("Value"=w191:bool)  [unwired: 2 in, 2 out]
              n193 = case shown="False" w191 {
                frame False {
                  w192 = FALSE ("As_Gas Active")
                  n194 = call "set_As_gas.vi"("Active"=w192, "As_Gas Flow"=0.0, "Gas In"=w192, "H2 Flush"=w192, "Run"=w192, "Remote"=w192) -> ()  [unwired: 10 in]
                }
                frame True {
                  w198 = TRUE ("As_Gas Active")
                  n195 = property on="AsH3 Run" class="Bool (strict)"() -> ("Value"=w194:bool)  [unwired: 2 in, 2 out]
                  n196 = property on="AsH3 Prep" class="Bool (strict)"() -> ("Value"=w195:bool)  [unwired: 2 in, 2 out]
                  n197 = And(x=w195, y=w194) -> (x .and. y?=w197:bool)
                  n198 = property on="Flow" class="DigNum (strict)"() -> ("Value"=w196:dbl)  [unwired: 2 in, 2 out]
                  n199 = call "set_As_gas.vi"("Active"=w198, "As_Gas Flow"=w196, "Gas In"=w198, "Run"=w197) -> ()  [unwired: 12 in]
                }
              }
            }
            frame #5 {
              n200 = property on="P bubbler Active" class="Bool (strict)"() -> ("Value"=w199:bool)  [unwired: 2 in, 2 out]
              n201 = case shown="False" w199 {
                frame False {
                  w200 = FALSE ("As_Gas Active")
                  n202 = call "set_P_Liq.vi"("flow 1"=0.0 ("As_Gas Flow"), "Remote"=w200, "Run"=w200, "Bubbler In"=w200, "Active"=w200) -> ()  [unwired: 5 in]
                }
                frame True {
                  w206 = TRUE ("As_Gas Active")
                  n203 = property on="Run" class="Bool (strict)"() -> ("Value"=w202:bool)  [unwired: 2 in, 2 out]
                  n204 = property on="Prep" class="Bool (strict)"() -> ("Value"=w203:bool)  [unwired: 2 in, 2 out]
                  n205 = And(x=w203, y=w202) -> (x .and. y?=w205:bool)
                  n206 = property on="Flow" class="DigNum (strict)"() -> ("Value"=w204:dbl)  [unwired: 2 in, 2 out]
                  n207 = call "set_P_Liq.vi"("flow 1"=w204, "Run"=w205, "Bubbler In"=w206, "Active"=w206) -> ()  [unwired: 6 in]
                }
              }
            }
          }
        }
        frame True {
        }
      }
    }
    frame "Run" {
      n208 = stacked-sequence {
        tunnel: w210 -> [_ w215 _ _]
        tunnel: w208 -> [w212 _ _ w266]
        tunnel: w209 -> [_ _ _ w265]
        tunnel: [_ _ _ w259] -> w207
        frame #0 {
          n209 = call "Get_Argument.vi"("Argument"="run_started", "Argument List"=w212) -> ("Enabled"=w211:bool)
          n210 = local write "run started"(w211) -> ()
        }
        frame #1 {
          n211 = property on="prep_time" class="DigNum (strict)"() -> ("Value"=w216:dbl)  [unwired: 2 in, 2 out]
          n212 = Greater Or Equal?(x=w215, y=w216) -> (x >= y?=w214:bool)
          n213 = local write "prep_done"(w214) -> ()
        }
        frame #2 {
          n214 = local read "run started"() -> (w218:bool)
          n215 = Not(x=w218) -> (.not. x?=w217:bool)
          n216 = stacked-sequence {
            tunnel: w217 -> [w220 w223 w229 w235 w241 w247 w253]
            frame #0 {
              n217 = case shown="True" w220 {
                tunnel: ["run: " "pre-run: "] -> w219
                frame False {
                }
                frame True {
                }
              }
              n218 = property on="Status Out" class="Str"("Value"=w219) -> ()  [unwired: 2 in, 2 out]
            }
            frame #1 {
              n219 = property on="Status Out" class="Str"() -> ("Value"=w228:string)  [unwired: 2 in, 2 out]
              n220 = call "flow_strings.vi"("string in"=w228, "is first in?"=TRUE, "name"="Al", "is prep?"=w223) -> ("string out"=w227:string, "is first out?"=w226:bool)  [unwired: 3 in]
              n221 = property on="Status Out" class="Str"("Value"=w227) -> ()  [unwired: 2 in, 2 out]
              n222 = property on="first" class="Bool (strict)"("Value"=w226) -> ()  [unwired: 2 in, 2 out]
            }
            frame #2 {
              n223 = property on="first" class="Bool (strict)"() -> ("Value"=w231:bool)  [unwired: 2 in, 2 out]
              n224 = property on="Status Out" class="Str"() -> ("Value"=w233:string)  [unwired: 2 in, 2 out]
              n225 = call "flow_strings.vi"("string in"=w233, "is first in?"=w231, "name"="Ga", "is prep?"=w229) -> ("string out"=w234:string, "is first out?"=w230:bool)  [unwired: 3 in]
              n226 = property on="Status Out" class="Str"("Value"=w234) -> ()  [unwired: 2 in, 2 out]
              n227 = property on="first" class="Bool (strict)"("Value"=w230) -> ()  [unwired: 2 in, 2 out]
            }
            frame #3 {
              n228 = property on="first" class="Bool (strict)"() -> ("Value"=w238:bool)  [unwired: 2 in, 2 out]
              n229 = property on="Status Out" class="Str"() -> ("Value"=w240:string)  [unwired: 2 in, 2 out]
              n230 = call "flow_strings.vi"("string in"=w240, "is first in?"=w238, "name"="In", "is prep?"=w235) -> ("string out"=w237:string, "is first out?"=w236:bool)  [unwired: 3 in]
              n231 = property on="Status Out" class="Str"("Value"=w237) -> ()  [unwired: 2 in, 2 out]
              n232 = property on="first" class="Bool (strict)"("Value"=w236) -> ()  [unwired: 2 in, 2 out]
            }
            frame #4 {
              n233 = property on="first" class="Bool (strict)"() -> ("Value"=w243:bool)  [unwired: 2 in, 2 out]
              n234 = property on="Status Out" class="Str"() -> ("Value"=w245:string)  [unwired: 2 in, 2 out]
              n235 = call "flow_strings.vi"("string in"=w245, "is first in?"=w243, "name"="PH3", "is prep?"=w241) -> ("string out"=w244:string, "is first out?"=w242:bool)  [unwired: 3 in]
              n236 = property on="Status Out" class="Str"("Value"=w244) -> ()  [unwired: 2 in, 2 out]
              n237 = property on="first" class="Bool (strict)"("Value"=w242) -> ()  [unwired: 2 in, 2 out]
            }
            frame #5 {
              n238 = property on="first" class="Bool (strict)"() -> ("Value"=w249:bool)  [unwired: 2 in, 2 out]
              n239 = property on="Status Out" class="Str"() -> ("Value"=w251:string)  [unwired: 2 in, 2 out]
              n240 = call "flow_strings.vi"("string in"=w251, "is first in?"=w249, "name"="AsH3", "is prep?"=w247) -> ("string out"=w248:string, "is first out?"=w250:bool)  [unwired: 3 in]
              n241 = property on="Status Out" class="Str"("Value"=w248) -> ()  [unwired: 2 in, 2 out]
              n242 = property on="first" class="Bool (strict)"("Value"=w250) -> ()  [unwired: 2 in, 2 out]
            }
            frame #6 {
              n243 = property on="first" class="Bool (strict)"() -> ("Value"=w256:bool)  [unwired: 2 in, 2 out]
              n244 = property on="Status Out" class="Str"() -> ("Value"=w258:string)  [unwired: 2 in, 2 out]
              n245 = call "flow_strings.vi"("string in"=w258, "is first in?"=w256, "name"="P liq", "is prep?"=w253) -> ("string out"=w255:string, "is first out?"=w254:bool)  [unwired: 3 in]
              n246 = property on="Status Out" class="Str"("Value"=w255) -> ()  [unwired: 2 in, 2 out]
              n247 = property on="first" class="Bool (strict)"("Value"=w254) -> ()  [unwired: 2 in, 2 out]
            }
          }
        }
        frame #3 {
          n248 = local read "prep_done"() -> (w263:bool)
          n249 = local read "run started"() -> (w262:bool)
          n250 = Not(x=w263) -> (.not. x?=w261:bool)
          n251 = Or(x=w261, y=w262) -> (x .or. y?=w260:bool)
          n252 = Or(x=w265, y=w260) -> (x .or. y?=w264:bool)
          n253 = case shown="False" w264 {
            tunnel: w266 -> [w268 w313]
            tunnel: [w267 w313] -> w259
            frame False {
              n254 = stacked-sequence {
                tunnel: [_ _ _ _ _ _ w310] -> w267
                tunnel: w268 -> [_ _ _ _ _ _ w309]
                frame #0 {
                  n255 = property on="Al Active" class="Bool (strict)"() -> ("Value"=w269:bool)  [unwired: 2 in, 2 out]
                  n256 = case shown="True" w269 {
                    frame False {
                      w270 = FALSE ("Al Active")
                      n257 = call "set_Al.vi"("ALMFC1"=0.0 ("Aluminum Flow"), "Remote"=w270, "Run"=w270, "Bubbler In"=w270, "Active"=w270) -> ()  [unwired: 5 out]
                    }
                    frame True {
                      w274 = TRUE ("Al Active")
                      n258 = property on="Al Flow" class="DigNum (strict)"() -> ("Value"=w273:dbl)  [unwired: 2 in, 2 out]
                      n259 = property on="Al Run" class="Bool (strict)"() -> ("Value"=w272:bool)  [unwired: 2 in, 2 out]
                      n260 = call "set_Al.vi"("ALMFC1"=w273, "Run"=w272, "Bubbler In"=w274, "Active"=w274) -> ()  [unwired: 1 in, 5 out]
                    }
                  }
                }
                frame #1 {
                  n261 = property on="Ga bubbler Active" class="Bool (strict)"() -> ("Value"=w275:bool)  [unwired: 2 in, 2 out]
                  n262 = case shown="True" w275 {
                    frame False {
                      w277 = FALSE ("Ga Active")
                      w276 = 0.0 ("Ga Flow 1")
                      n263 = call "set_Ga.vi"("Active"=w277, "GAMFC3"=w276, "GAMFC2"=w276, "GAMFC1"=w276, "Bubbler In"=w277, "H2 Dilute"=w277, "Run"=w277, "Remote"=w277) -> ()  [unwired: 8 out]
                    }
                    frame True {
                      w283 = TRUE ("Ga Active")
                      n264 = property on="MFC2 flow" class="DigNum (strict)"() -> ("Value"=w279:dbl)  [unwired: 2 in, 2 out]
                      n265 = property on="MFC3 flow" class="DigNum (strict)"() -> ("Value"=w278:dbl)  [unwired: 2 in, 2 out]
                      n266 = property on="Run" class="Bool (strict)"() -> ("Value"=w282:bool)  [unwired: 2 in, 2 out]
                      n267 = property on="MFC1 flow" class="DigNum (strict)"() -> ("Value"=w280:dbl)  [unwired: 2 in, 2 out]
                      n268 = property on="Dilution" class="Bool (strict)"() -> ("Value"=w281:bool)  [unwired: 2 in, 2 out]
                      n269 = call "set_Ga.vi"("Active"=w283, "GAMFC3"=w278, "GAMFC2"=w279, "GAMFC1"=w280, "Bubbler In"=w283, "H2 Dilute"=w281, "Run"=w282, "Remote"=w283) -> ()  [unwired: 8 in]
                    }
                  }
                }
                frame #2 {
                  n270 = property on="In bubbler Active" class="Bool (strict)"() -> ("Value"=w284:bool)  [unwired: 2 in, 2 out]
                  n271 = case shown="True" w284 {
                    frame False {
                      w286 = FALSE ("In Remote")
                      n272 = call "set_In.vi"("INMFC1"=0.0 ("Indium Flow"), "Remote"=w286, "Run"=w286, "Bubbler In"=w286, "Active"=w286) -> ()  [unwired: 5 out]
                    }
                    frame True {
                      w289 = TRUE ("In Run")
                      n273 = property on="Run" class="Bool (strict)"() -> ("Value"=w287:bool)  [unwired: 2 in, 2 out]
                      n274 = property on="In Flow" class="DigNum (strict)"() -> ("Value"=w288:dbl)  [unwired: 2 in, 2 out]
                      n275 = call "set_In.vi"("INMFC1"=w288, "Run"=w287, "Bubbler In"=w289, "Active"=w289) -> ()  [unwired: 1 in, 5 out]
                    }
                  }
                }
                frame #3 {
                  n276 = property on="P gas Active" class="Bool (strict)"() -> ("Value"=w290:bool)  [unwired: 2 in, 2 out]
                  n277 = case shown="False" w290 {
                    frame False {
                      w291 = FALSE ("P_Gas Active")
                      n278 = call "set_P_gas.vi"("Run"=w291, "Gas In"=w291, "Active"=w291, "P_Gas Remote"=w291, "H2 Flush"=w291, "P_Gas Flow"=0.0) -> ()
                    }
                    frame True {
                      n279 = property on="Run" class="Bool (strict)"() -> ("Value"=w294:bool)  [unwired: 2 in, 2 out]
                      n280 = property on="Flow" class="DigNum (strict)"() -> ("Value"=w295:dbl)  [unwired: 2 in, 2 out]
                      n281 = call "set_P_gas.vi"("Run"=w294, "Gas In"=TRUE, "Active"=TRUE ("P_Gas Active"), "P_Gas Flow"=w295) -> ()  [unwired: 2 in]
                    }
                  }
                }
                frame #4 {
                  n282 = property on="As gas Active" class="Bool (strict)"() -> ("Value"=w297:bool)  [unwired: 2 in, 2 out]
                  n283 = case shown="True" w297 {
                    frame False {
                      w298 = FALSE ("As_Gas Active")
                      n284 = call "set_As_gas.vi"("Active"=w298, "As_Gas Flow"=0.0, "Gas In"=w298, "H2 Flush"=w298, "Run"=w298, "Remote"=w298) -> ()  [unwired: 10 in]
                    }
                    frame True {
                      w302 = TRUE ("As_Gas Active")
                      n285 = property on="AsH3 Run" class="Bool (strict)"() -> ("Value"=w301:bool)  [unwired: 2 in, 2 out]
                      n286 = property on="Flow" class="DigNum (strict)"() -> ("Value"=w300:dbl)  [unwired: 2 in, 2 out]
                      n287 = call "set_As_gas.vi"("Active"=w302, "As_Gas Flow"=w300, "Gas In"=w302, "Run"=w301) -> ()  [unwired: 12 in]
                    }
                  }
                }
                frame #5 {
                  n288 = property on="P bubbler Active" class="Bool (strict)"() -> ("Value"=w303:bool)  [unwired: 2 in, 2 out]
                  n289 = case shown="True" w303 {
                    frame False {
                      w305 = FALSE ("In Remote")
                      n290 = call "set_P_Liq.vi"("flow 1"=0.0 ("Indium Flow"), "Remote"=w305, "Run"=w305, "Bubbler In"=w305, "Active"=w305) -> ()  [unwired: 5 in]
                    }
                    frame True {
                      w308 = TRUE ("In Run")
                      n291 = property on="Flow" class="DigNum (strict)"() -> ("Value"=w307:dbl)  [unwired: 2 in, 2 out]
                      n292 = property on="Run" class="Bool (strict)"() -> ("Value"=w306:bool)  [unwired: 2 in, 2 out]
                      n293 = call "set_P_Liq.vi"("flow 1"=w307, "Run"=w306, "Bubbler In"=w308, "Active"=w308) -> ()  [unwired: 6 in]
                    }
                  }
                }
                frame #6 {
                  n294 = call "Set_Argument.vi"("Enable"=TRUE, "Argument"="run_started", "Argument List In"=w309) -> ("Argument List Out"=w310:string[])
                }
              }
            }
            frame True {
            }
          }
        }
      }
    }
    frame "End" {
    }
    frame "Idle" {
    }
  }
  "Argument List Out" <- w10
